vi "RestartApp.vi"   [LabVIEW 2017]
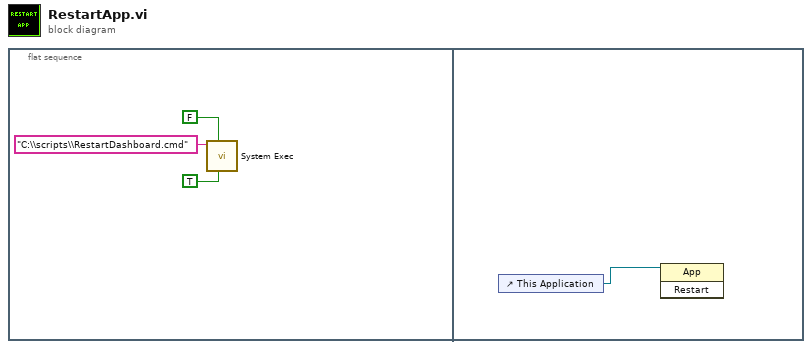
[diagram p0: block diagram]
diagram:
  n1 = flat-sequence {
    frame #0 {
      n2 = call <vilib>:"System Exec.vi"("run minimized? (F)"=TRUE, "wait until completion? (T)"=FALSE, "command line"="C:\\scripts\\RestartDashboard.cmd") -> ()  [unwired: 5 in, 4 out]
    }
    frame #1 {
      n3 = control-ref of="This Application"() -> (w4:refnum<vi>)
      n4 = invoke class="App" method="Restart"(reference=w4) -> ()  [unwired: 2 in, 3 out]
    }
  }
